vi "Launch Edit Popup.vi"(8 "error in":errorcluster, 10 "Data":string, 11 "Selected Tag":string) -> (0 "error out":errorcluster, 3 "Data Out":string)   [LabVIEW 2019]
doc: "All Rights Reserved © 2017 SyncSols"
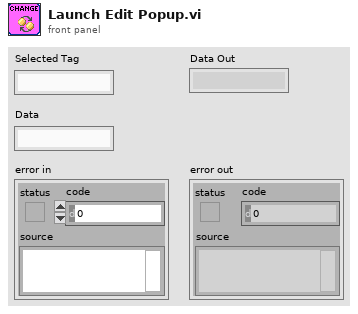
[diagram p1: front panel]
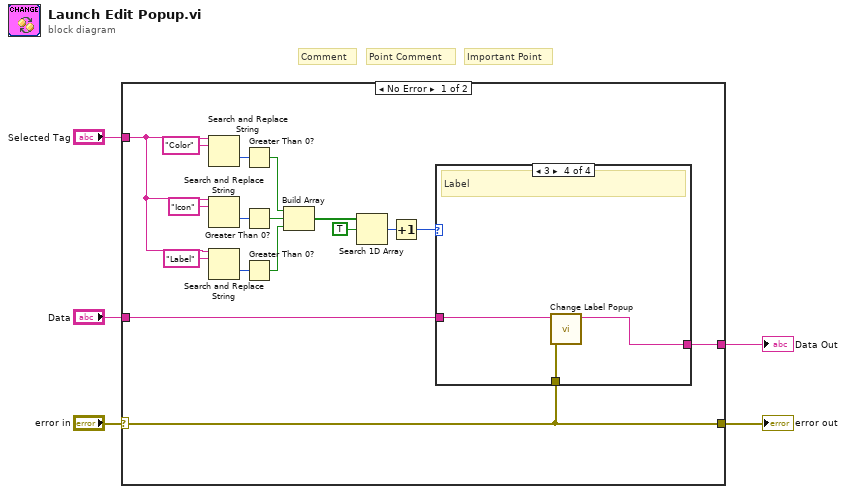
[diagram p0: block diagram]
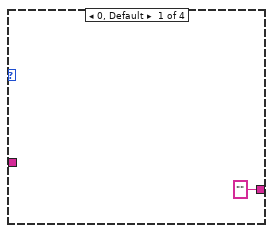
[diagram p2: hidden frame]
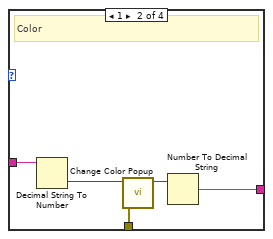
[diagram p3: hidden frame]
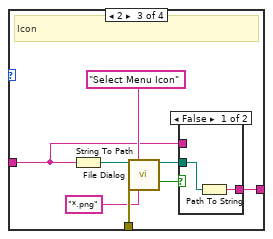
[diagram p4: hidden frame]
diagram:
  # "Important Point"
  # "Point Comment"
  # "Comment"
  n1 = case shown="No Error" "error in" {
    selector: "error in" -> [w7 w43]
    tunnel: [w7 w43] -> w5
    tunnel: "Selected Tag" -> [w16 _]
    tunnel: "Data" -> [w8 _]
    tunnel: [w6 _] -> w1
    frame No Error {
      n2 = Search and Replace String(input string=w16, search string="Color") -> (offset past replacement=w21:i32)  [unwired: 6 in, 3 out]
      n3 = Search and Replace String(input string=w16, search string="Icon") -> (offset past replacement=w20:i32)  [unwired: 6 in, 3 out]
      n4 = Search and Replace String(input string=w16, search string="Label") -> (offset past replacement=w17:i32)  [unwired: 6 in, 3 out]
      n5 = Greater Than 0?(x=w21) -> (x > 0?=w14:bool)
      n6 = Greater Than 0?(x=w20) -> (x > 0?=w15:bool)
      n7 = Greater Than 0?(x=w17) -> (x > 0?=w13:bool)
      n8 = Build Array(w14, w15, w13) -> (w12:bool[])
      n9 = Search 1D Array(1D array=w12, element=TRUE) -> (index of element=w10:i32)  [unwired: 1 in]
      n10 = Increment(x=w10) -> (x+1=w9:i32)
      n11 = case shown="3" w9 {
        tunnel: w8 -> [_ w28 w29 w41]
        tunnel: w7 -> [_ w26 w36 w42]
        tunnel: ["" ("Label Out") w24 w32 w40] -> w6
        frame 0, Default {
        }
        frame 1 {
          # "Color"
          n12 = Decimal String To Number(string=w28) -> (number=w27:i32)  [unwired: 2 in, 1 out]
          n13 = call "Change Color Popup.vi"("error in"=w26, "Color Value In"=w27) -> ("Color Value Out"=w25:u32)  [unwired: 8 in, 1 out]
          n14 = Number To Decimal String(number=w25) -> (decimal integer string=w24:string)  [unwired: 1 in]
        }
        frame 2 {
          # "Icon"
          n15 = String To Path(string=w29) -> (path=w35:path)
          n16 = call "File Dialog"("start path"=w35, "prompt"="Select Menu Icon", "error in"=w36, "pattern (all files)"="*.png") -> ("selected path"=w31:path, "cancelled"=w30:bool)  [unwired: 8 in, 2 out]
          n17 = case shown="False" w30 {
            tunnel: [w38 w39] -> w32
            tunnel: w31 -> [w37 _]
            tunnel: w29 -> [_ w39]
            frame False {
              n18 = Path To String(path=w37) -> (string=w38:string)
            }
            frame True {
            }
          }
        }
        frame 3 {
          # "Label"
          n19 = call "Change Label Popup.vi"("error in"=w42, "Label In"=w41) -> ("Label Out"=w40:string)  [unwired: 8 in, 1 out]
        }
      }
    }
    frame Error {
    }
  }
  "error out" <- w5
  "Data Out" <- w1
